vi "Add Alias_Alias Folder.vi"(8 "error in (no error)":errorcluster, 10 "Alias Settings":T1, 11 "Aliases Folder Ref":refnum<k24>) -> (0 "error out":errorcluster, 3 "Aliases Folder Ref Out":refnum<k24>)   [LabVIEW 2019, in "Simple SysDef API.lvlib"]
uses:
  <userlib>/SimpleSysDef/Simple SysDef API.lvlib
  NationalInstruments.VeriStand.SystemDefinitionAPI
  <userlib>/SimpleSysDef/_SubVIs/Add Alias_Alias Settings.ctl
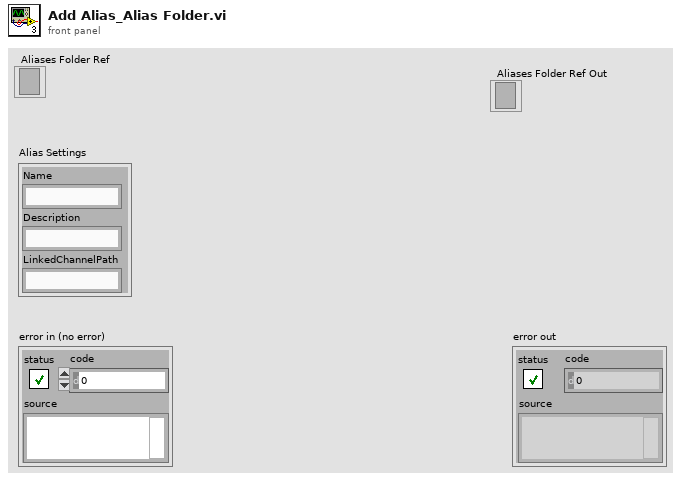
[diagram p1: front panel]
types:
  T1 = typedef "Simple SysDef API.lvlib/Add Alias_Alias Settings.ctl" = cluster{"Name":string, "Description":string, "LinkedChannelPath":string}
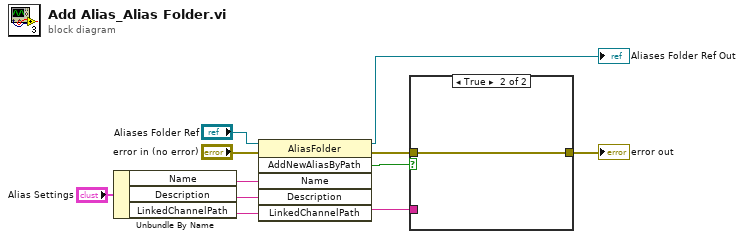
[diagram p0: block diagram]
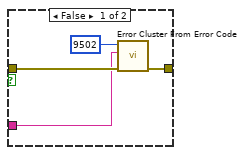
[diagram p2: hidden frame]
diagram:
  n1 = Unbundle By Name("Alias Settings") -> ("Name"=w4:string, "Description"=w3:string, "LinkedChannelPath"=w2:string)
  n2 = invoke class="AliasFolder" method="AddNewAliasByPath"(reference="Aliases Folder Ref", error in="error in (no error)", "Name"=w4, "Description"=w3, "LinkedChannelPath"=w2) -> (reference out=→"Aliases Folder Ref Out":refnum<k24>, error out=w7:errorcluster, "AddNewAliasByPath"=w8:bool)  [unwired: 1 in, 3 out]
  n3 = case shown="True" w8 {
    tunnel: w7 -> [w14 w15]
    tunnel: [w13 w15] -> w6
    tunnel: w2 -> [w11 _]
    frame False {
      n4 = call <userlib>:"Error Cluster From Error Code.vi"("error in (no error)"=w14, "error message (\"\")"=w11, "error code (0)"=9502) -> ("error out"=w13:errorcluster)  [unwired: 6 in]
    }
    frame True {
    }
  }
  "error out" <- w6
